vi "Read_Joystick.vi"(8 "error in (no error)":errorcluster, 11 "Teleop_Lift in":refnum<class "Teleop_Lift.lvclass">) -> (0 "error out":errorcluster, 3 "Teleop_Lift out":refnum<class "Teleop_Lift.lvclass">)   [LabVIEW 2018, in "Teleop_Lift.lvclass"]
uses:
  Teleop_Lift.lvclass
panel:
  in  "Autonomous?":bool=TRUE
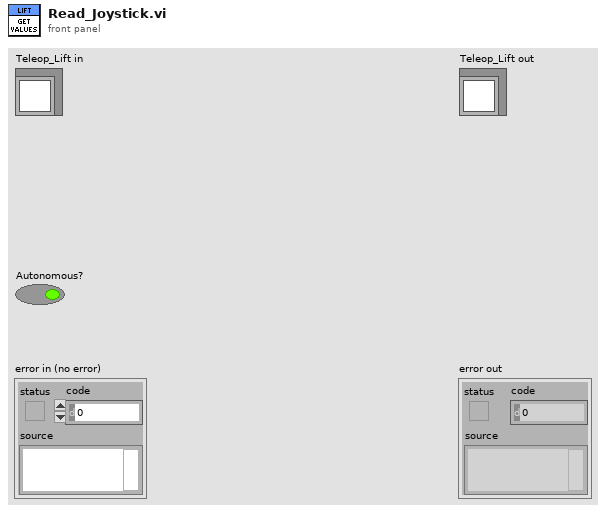
[diagram p1: front panel]
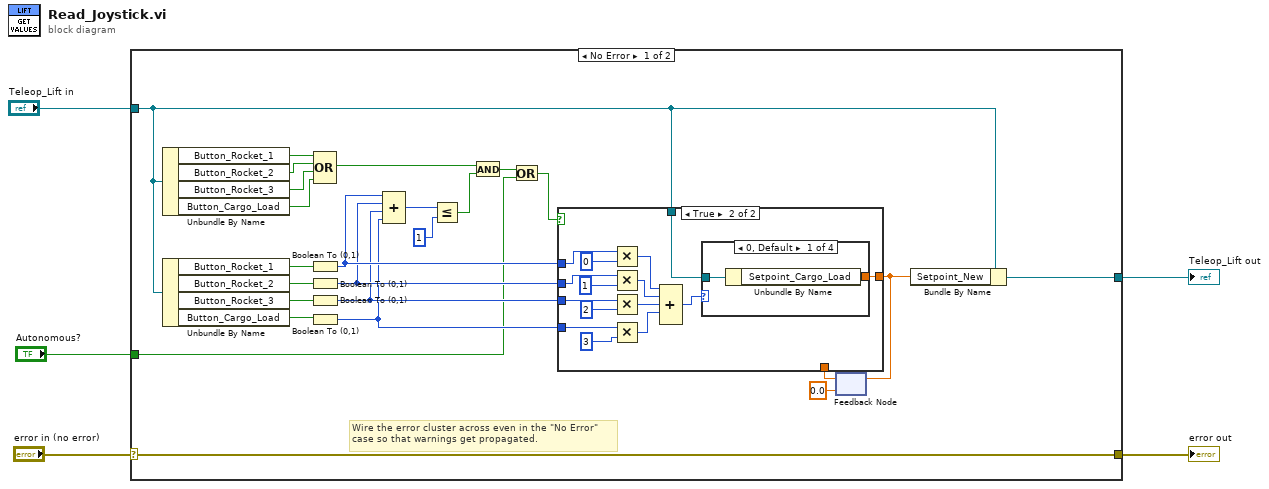
[diagram p0: block diagram]
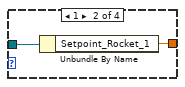
[diagram p3: hidden frame]
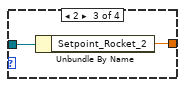
[diagram p4: hidden frame]
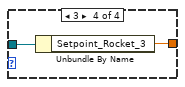
[diagram p5: hidden frame]
diagram:
  n1 = case shown="No Error" "error in (no error)" {
    selector: "error in (no error)" -> [w30 w56]
    tunnel: [w30 w56] -> w4
    tunnel: [w12 w55] -> w2
    tunnel: "Teleop_Lift in" -> [w14 w55]
    tunnel: "Autonomous?" -> [w6 _]
    frame No Error {
      # "Wire the error cluster across even in the \"No Error\"\ncase so that warnings get propagated."
      n2 = Unbundle By Name(w14) -> ("Button_Rocket_1"=w29:bool, "Button_Rocket_2"=w28:bool, "Button_Rocket_3"=w27:bool, "Button_Cargo_Load"=w11:bool)
      n3 = Unbundle By Name(w14) -> ("Button_Rocket_1"=w26:bool, "Button_Rocket_2"=w25:bool, "Button_Rocket_3"=w24:bool, "Button_Cargo_Load"=w10:bool)
      n4 = Boolean To (0,1)(Boolean=w26) -> (0, 1=w19:i16)
      n5 = Boolean To (0,1)(Boolean=w25) -> (0, 1=w18:i16)
      n6 = Boolean To (0,1)(Boolean=w24) -> (0, 1=w17:i16)
      n7 = Boolean To (0,1)(Boolean=w10) -> (0, 1=w9:i16)
      n8 = Compound Arithmetic op=OR(w29, w28, w27, w11) -> (w20:bool)
      n9 = Compound Arithmetic op=ADD(w19, w18, w17, w9) -> (w22:i16)
      n10 = Less Or Equal?(x=w22, y=i16 1) -> (x <= y?=w21:bool)
      n11 = And(x=w20, y=w21) -> (x .and. y?=w8:bool)
      n12 = Or(x=w8, y=w6) -> (x .or. y?=w7:bool)
      n13 = feedback #1(0.0 ("Setpoint_High")) -> (w16:dbl)
      n14 = case shown="True" w7 {
        tunnel: w17 -> [_ w42]
        tunnel: w18 -> [_ w40]
        tunnel: w19 -> [_ w38]
        tunnel: [w31 w36] -> w13
        tunnel: w14 -> [_ w35]
        tunnel: w16 -> [w31 _]
        tunnel: w9 -> [_ w34]
        frame False {
        }
        frame True {
          n15 = Multiply(x=w38, y=0) -> (x*y=w44:i32)
          n16 = Multiply(x=w40, y=1) -> (x*y=w46:i32)
          n17 = Multiply(x=w42, y=2) -> (x*y=w45:i32)
          n18 = Multiply(x=w34, y=3) -> (x*y=w32:i32)
          n19 = Compound Arithmetic op=ADD(w44, w46, w45, w32) -> (w37:i32)  [unwired: 1 in]
          n20 = case shown="0, Default" w37 {
            tunnel: [w47 w49 w51 w53] -> w36
            tunnel: w35 -> [w48 w50 w52 w54]
            frame 0, Default {
              n21 = Unbundle By Name(w48) -> ("Setpoint_Cargo_Load"=w47:dbl)
            }
            frame 1 {
              n22 = Unbundle By Name(w50) -> ("Setpoint_Rocket_1"=w49:dbl)
            }
            frame 2 {
              n23 = Unbundle By Name(w52) -> ("Setpoint_Rocket_2"=w51:dbl)
            }
            frame 3 {
              n24 = Unbundle By Name(w54) -> ("Setpoint_Rocket_3"=w53:dbl)
            }
          }
        }
      }
      n25 = feedback-in #1(w13) -> ()
      n26 = Bundle By Name(cluster=w14, "Setpoint_New"=w13) -> (w12:refnum<class "Teleop_Lift.lvclass">)
    }
    frame Error {
    }
  }
  "error out" <- w4
  "Teleop_Lift out" <- w2
